vi "Generate Linear Accel Segment.vi"(0 "Speeds in":T1={"maxV (fps)"=20.0, "Accel Limit (fps^2)"=20.0, "Initial V (fps)"=0.0, "Sample Period (s)"=0.02, "Jerk Limit (fps^3)"=0.0, "Distances"=[]}, 1 "Initial Acceleration":dbl format="%#_13g", 5 "Stoopid V":dbl=20.0, 7 "Velocities":dbl[](array[numeric]), 9 "Linear Info":T2, 11 "Max Robot Speed":dbl format="%#_13g", 12 "Index":i32, 14 "Stoopid Overlap distance":dbl min=0.0) -> (3 "Final Acceleration":dbl, 4 "Speeds out":T1={"maxV (fps)"=20.0, "Accel Limit (fps^2)"=20.0, "Initial V (fps)"=0.0, "Sample Period (s)"=0.02, "Jerk Limit (fps^3)"=0.0, "Distances"=[]}, 6 "Trajectory Segment":T3, 10 "Final Position":cluster{dbl, dbl, dbl}, 15 "Valid":bool)   [LabVIEW 2025]
uses:
  Types/Speeds.ctl
panel:
  out "Waveform Graph":dbl[][](graph)
  out "XY Graph":cluster{dbl, dbl}[](graph)
  out "Segment Time (s)":dbl
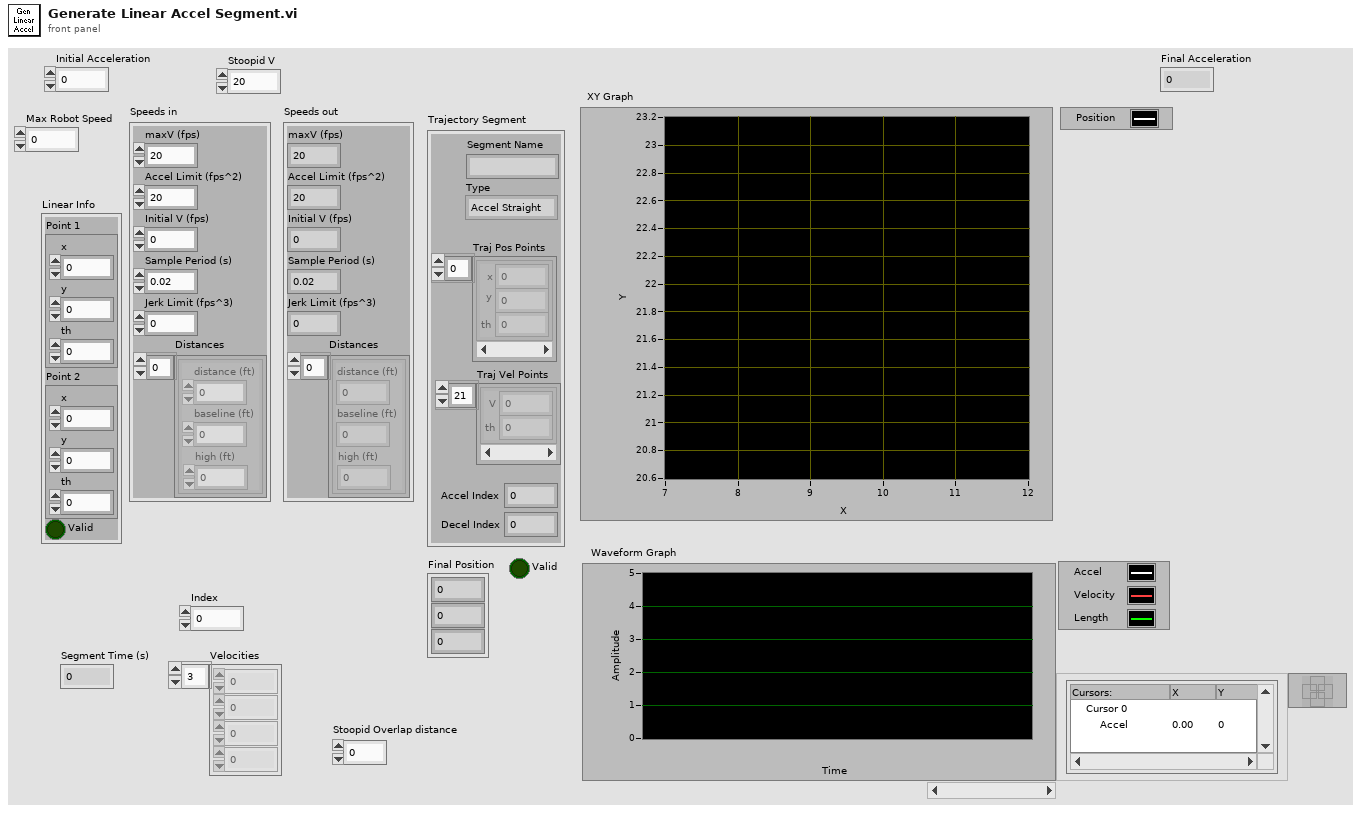
[diagram p1: front panel]
types:
  T1 = typedef "Speeds.ctl" = cluster{"maxV (fps)":dbl, "Accel Limit (fps^2)":dbl, "Initial V (fps)":dbl, "Sample Period (s)":dbl, "Jerk Limit (fps^3)":dbl, "Distances":cluster{"distance (ft)":dbl, "baseline (ft)":dbl, "high (ft)":dbl}[]}
  T2 = cluster{"Point 1":cluster{"x":dbl, "y":dbl, "th":dbl}, "Point 2":cluster{"x":dbl, "y":dbl, "th":dbl}, "Valid":bool}
  T3 = cluster{"Segment Name":string, "Type":enum16{"Accel Straight", "Const Straight", "Blend", "Circle"}, "Traj Pos Points":cluster{"x":dbl, "y":dbl, "th":dbl}[], "Traj Vel Points":cluster{"V":dbl, "th":dbl}[], "Accel Index":i32, "Decel Index":i32}
  T4 = enum16{"Accel Straight", "Const Straight", "Blend", "Circle"}
  T5 = cluster{"Accel Limit (fps^2)":dbl, "Jerk Limit (fps^3)":dbl}
  T6 = cluster{"distance (ft)":dbl, "dist baseline jerk":dbl, "dist of high Jerk":dbl}[]
  T7 = cluster{"Initial Acceleration":dbl, "Initial V (fps)":dbl}
  T8 = cluster{string, "Type":enum16{"Accel Straight", "Const Straight", "Blend", "Circle"}, cluster{dbl, dbl, dbl}[], cluster{"velocity":dbl, dbl}[], "Accel Index":i32, "Decel Index":i32}
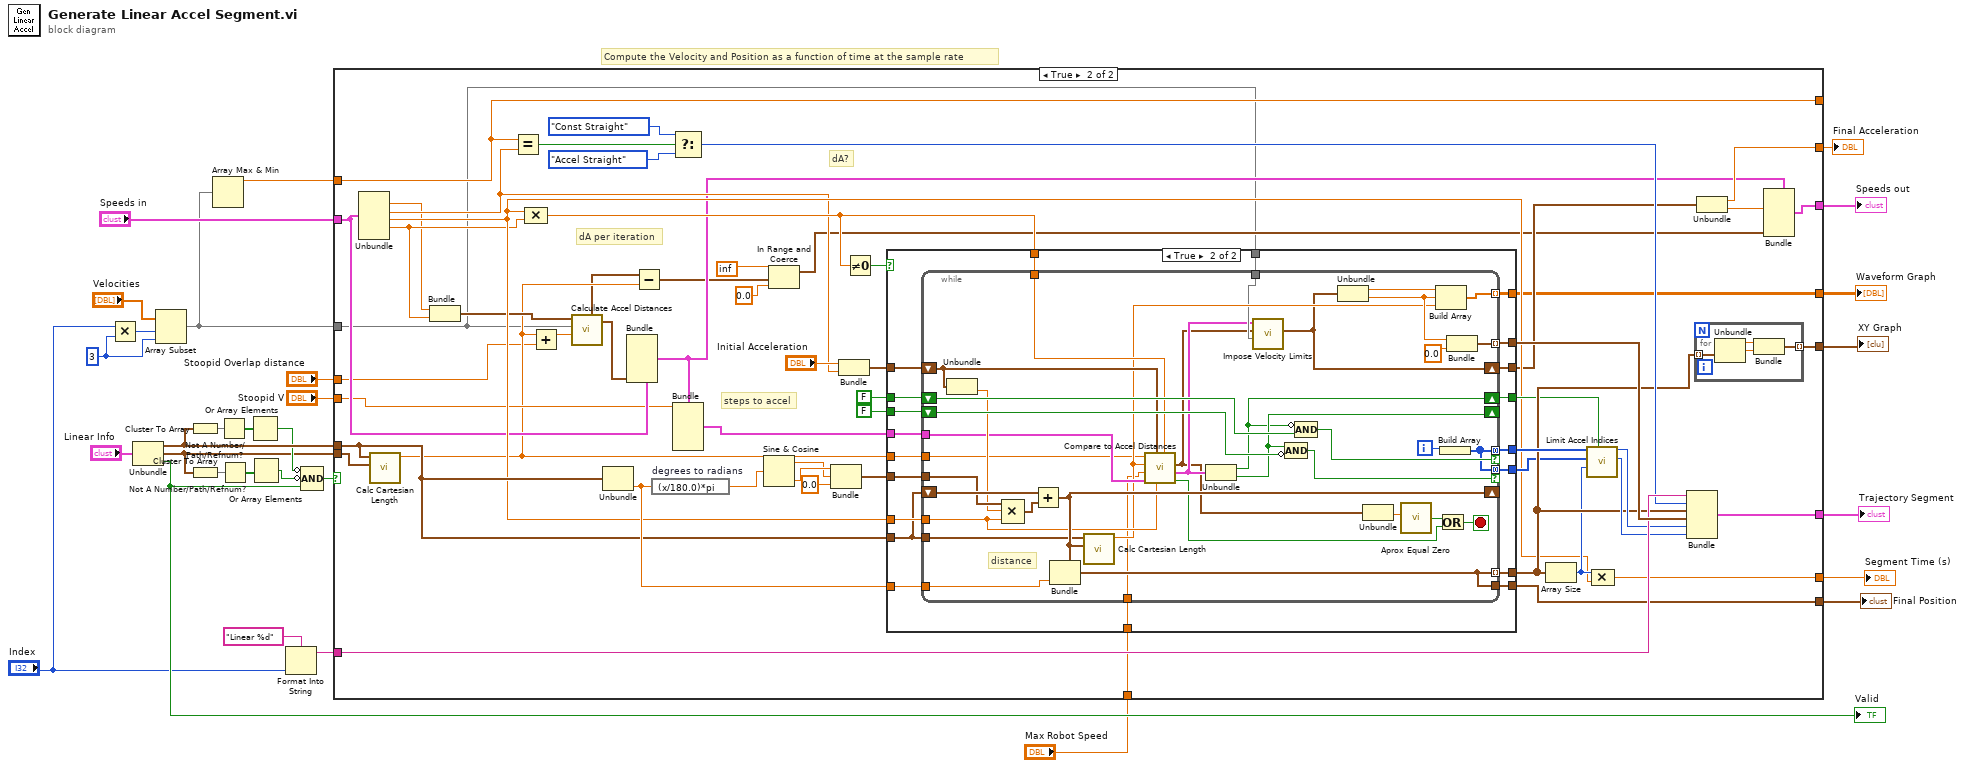
[diagram p0: block diagram]
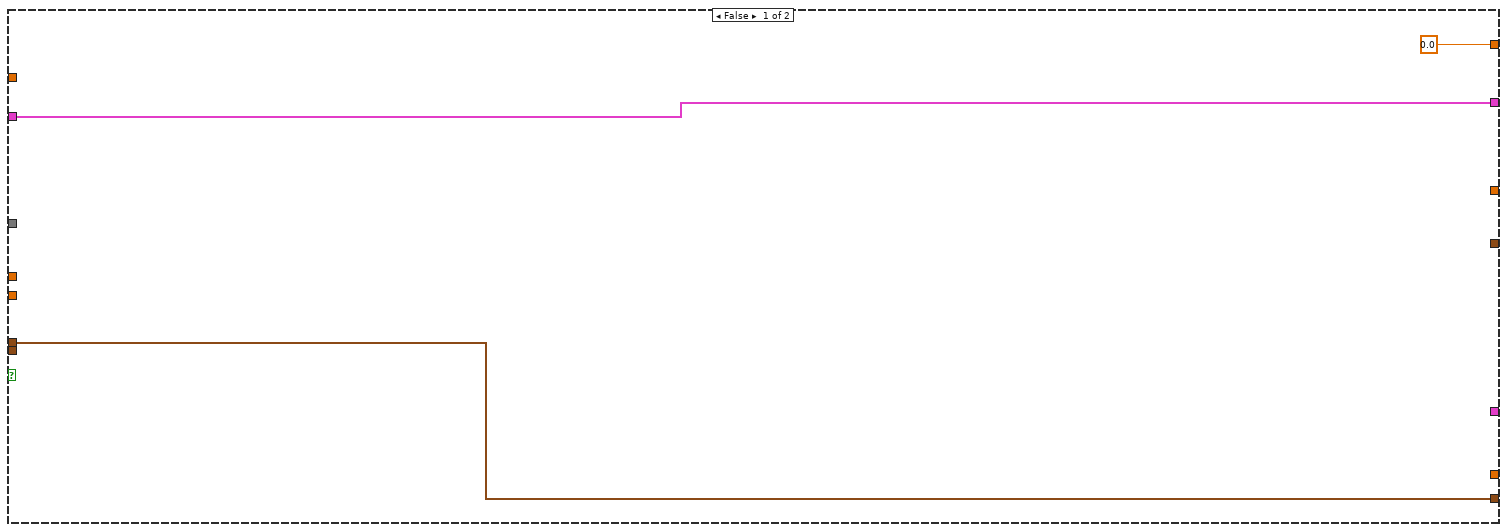
[diagram p2: hidden frame]
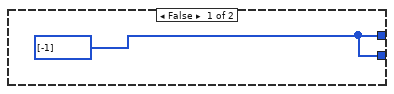
[diagram p3: hidden frame]
diagram:
  w7 = 3
  # "Compute the Velocity and Position as a function of time at the sample rate"
  n1 = Multiply(x="Index", y=w7) -> (x*y=w9:i32)
  n2 = Unbundle("Linear Info") -> ("Point 1"=w19:cluster{"x":dbl, "y":dbl, "th":dbl}, "Point 2"=w14:cluster{"x":dbl, "y":dbl, "th":dbl}, "Valid"=w20:bool)
  "Valid" <- w20
  n3 = Array Subset(array="Velocities", index=w9, length=w7) -> (w5:dbl[])
  n4 = Cluster To Array(cluster=w19) -> (array=w18:dbl[])
  n5 = Cluster To Array(cluster=w14) -> (array=w15:dbl[])
  n6 = Array Max & Min(array=w5) -> (max value=w4:dbl)  [unwired: 3 out]
  n7 = Not A Number/Path/Refnum?(number/path/refnum=w18) -> (NaN/Path/Refnum?=w17:bool[])
  n8 = Not A Number/Path/Refnum?(number/path/refnum=w15) -> (NaN/Path/Refnum?=w13:bool[])
  n9 = Or Array Elements(Boolean array=w17) -> (logical OR=w16:bool)
  n10 = Or Array Elements(Boolean array=w13) -> (logical OR=w12:bool)
  n11 = Format Into String(format string="Linear %d", "Index") -> (resulting string=w22:string)  [unwired: 2 in, 1 out]
  n12 = Compound Arithmetic op=AND(invert w16, invert w12, w20) -> (w21:bool)
  n13 = case shown="True" w21 {
    tunnel: [_ w90] -> w30
    tunnel: w22 -> [_ w84]
    tunnel: [_ w80] -> w29
    tunnel: [w32 w79] -> w28
    tunnel: [_ w76] -> w27
    tunnel: "Speeds in" -> [w33 w49]
    tunnel: [w33 w75] -> w25
    tunnel: w19 -> [w32 w70]
    tunnel: w14 -> [_ w73]
    tunnel: [_ w54] -> w11
    tunnel: [0.0 w53] -> w10
    tunnel: w5 -> [_ w35]
    tunnel: w4 -> [_ w48]
    tunnel: "Stoopid V" -> [_ w45]
    tunnel: [_ w48] -> _
    tunnel: "Stoopid Overlap distance" -> [_ w39]
    tunnel: "Max Robot Speed" -> [_ w34]
    frame False {
    }
    frame True {
      # "dA?"
      # "steps to accel"
      # "dA per iteration"
      n14 = Unbundle(w49) -> ("Accel Limit (fps^2)"=w51:dbl, "Initial V (fps)"=w58:dbl, "Sample Period (s)"=w60:dbl, "Jerk Limit (fps^3)"=w52:dbl)  [unwired: 2 out]
      n15 = call "Calc Cartesian Length.vi"("Point 2"=w73, "Point 1"=w70) -> ("Length (f)"=w44:dbl)  [unwired: 8 in, 1 out]
      n16 = Bundle("Accel Limit (fps^2)"=w51, "Jerk Limit (fps^3)"=w52) -> (w50:T5)  [unwired: 1 in]
      n17 = Equal?(x=w48, y=w58) -> (x = y?=w74:bool)
      n18 = Compound Arithmetic op=MULTIPLY(w60, w52) -> (w72:dbl)
      n19 = Add(x=w44, y=w39) -> (x+y=w38:dbl)
      n20 = call "Calculate Accel Distances.vi"("Length (f)"=w38, "Velocities"=w35, "Limits"=w50) -> ("Distances"=w37:T6, "Const V Dist"=w36:T6)  [unwired: 7 in]
      n21 = Unbundle(w70) -> ("th"=w78:dbl)  [unwired: 2 out]
      n22 = Bundle(cluster=w49, "Distances"=w37) -> (w47:T1)  [unwired: 5 in]
      n23 = Subtract(x=w36, y=w44) -> (x-y=w41:T6)
      n24 = expression code="(x/180.0)*pi" "degrees to radians"(w78) -> (w77:dbl)
      n25 = Select(t=T4."Const Straight" ("Type"), s=w74, f=T4."Accel Straight" ("Type")) -> (s? t:f=w81:T4)
      n26 = Bundle(cluster=w47, "maxV (fps)"=w45) -> (w46:T1)  [unwired: 5 in]
      n27 = Sine & Cosine(0:w77) -> (1:w85:dbl, 2:w86:dbl)
      n28 = In Range and Coerce(upper limit=inf, x=w41, lower limit=0.0) -> (coerced(x)=w40:T6)  [unwired: 1 out]
      n29 = Bundle(w86, w85, 0.0) -> (w88:cluster{dbl, dbl, dbl})  [unwired: 1 in]
      n30 = Bundle("Initial Acceleration"="Initial Acceleration", "Initial V (fps)"=w58) -> (w57:T7)  [unwired: 1 in]
      n31 = Not Equal To 0?(x=w72) -> (x != 0?=w71:bool)
      n32 = case shown="True" w71 {
        tunnel: [_ w115] -> w89
        tunnel: w88 -> [_ w114]
        tunnel: [_ w113] -> w79
        tunnel: w78 -> [_ w112]
        tunnel: [_ w111] -> w64
        tunnel: [_ w110] -> w56
        tunnel: w72 -> [_ w109]
        tunnel: w60 -> [_ w108]
        tunnel: w70 -> [_ w107]
        tunnel: FALSE -> [_ w106]
        tunnel: [w95 w105] -> w67
        tunnel: w46 -> [_ w104]
        tunnel: FALSE -> [_ w103]
        tunnel: [w95 w102] -> w63
        tunnel: [_ w101] -> w61
        tunnel: w57 -> [_ w100]
        tunnel: [_ w99] -> w54
        tunnel: w44 -> [_ w98]
        tunnel: w35 -> [_ w97]
        tunnel: w34 -> [_ w96]
        frame False {
          w95 = i32[] [-1]
        }
        frame True {
          n33 = while {
            tunnel: [w143] -> w111 mode=indexing
            tunnel: w109 -> [w130]
            shift-right: [w117] -> w110
            shift-left: w100 -> [w133]
            tunnel: [w149] -> w115 mode=indexing
            tunnel: w108 -> [w127]
            tunnel: w114 -> [w147]
            tunnel: w112 -> [w150]
            tunnel: [w143] -> w113
            shift-right: [w145] -> _
            shift-left: w107 -> [w148]
            tunnel: w107 -> [w144]
            shift-right: [w129] -> w101
            shift-left: w106 -> [w141]
            tunnel: [w138] -> w105 mode=concatenating if=w140
            tunnel: w104 -> [w126]
            shift-right: [w132] -> _
            shift-left: w103 -> [w139]
            tunnel: [w138] -> w102 mode=concatenating if=w137
            tunnel: [w128] -> w99 mode=indexing
            tunnel: w98 -> [w122]
            tunnel: w97 -> [w120]
            tunnel: w96 -> [w116]
            i -> [w142]
            stop <- w136 stop-if-true
            # "distance"
            n34 = Unbundle(w133) -> ("Initial V (fps)"=w134:dbl)  [unwired: 1 out]
            n35 = Compound Arithmetic op=MULTIPLY(w147, w134, w127) -> (w146:cluster{dbl, dbl, dbl})
            n36 = Add(x=w148, y=w146) -> (x+y=w145:cluster{dbl, dbl, dbl})
            n37 = Bundle(cluster=w145, w150) -> (w143:cluster{dbl, dbl, dbl})  [unwired: 2 in]
            n38 = call "Calc Cartesian Length.vi"("Point 2"=w145, "Point 1"=w144) -> ("Length (f)"=w123:dbl)  [unwired: 8 in, 1 out]
            n39 = call "Compare to Accel Distances.vi"("dA"=w130, "Sample Period (s)"=w127, "Values"=w133, "Speeds in"=w126, "Max Robot Speed"=w116, "Current  Length"=w123, "Total Segment Length"=w122) -> ("End Loop"=w121:bool, "Ends"=w119:cluster{"Accel End":bool, "Decel End":bool}, "Values out"=w118:cluster{"accel":dbl, "velocity":dbl})  [unwired: 1 in, 1 out]
            n40 = Unbundle(w119) -> ("Accel End"=w129:bool, "Decel End"=w132:bool)
            n41 = call "Impose Velocity Limits.vi"("Array"=w120, "Values in"=w118, "Ends"=w119) -> ("Values out"=w117:cluster{"accel":dbl, "velocity":dbl})  [unwired: 8 in]
            n42 = Compound Arithmetic op=AND(w132, invert w139) -> (w137:bool)
            n43 = Compound Arithmetic op=AND(invert w129, w141) -> (w140:bool)
            n44 = Unbundle(w117) -> ("accel"=w124:dbl, "velocity"=w125:dbl)
            n45 = Unbundle(w118) -> ("velocity"=w131:dbl)  [unwired: 1 out]
            n46 = call "Aprox Equal Zero.vi"("x"=w131) -> ("Boolean"=w135:bool)  [unwired: 10 in]
            n47 = Build Array(w124, w125, w123) -> (w128:dbl[])
            n48 = Or(x=w135, y=w121) -> (x .or. y?=w136:bool)
            n49 = Build Array(w142) -> (w138:i32[])
            n50 = Bundle("velocity"=w125, 0.0) -> (w149:cluster{"velocity":dbl, dbl})  [unwired: 1 in]
          }
        }
      }
      n51 = Array Size(array=w64) -> (size(s)=w62:i32)
      n52 = call "Limit Accel Indices.vi"("Last Accel"=w61, "Size"=w62, "Decel"=w63, "Accel"=w67) -> ("Decel Index"=w66:i32, "Accel Index"=w68:i32)  [unwired: 6 in]
      n53 = Compound Arithmetic op=MULTIPLY(w62, w60) -> (w80:dbl)
      n54 = Bundle(w84, "Type"=w81, w64, w89, "Accel Index"=w68, "Decel Index"=w66) -> (w90:T8)  [unwired: 1 in]
      n55 = for {
        tunnel: w64 -> [w94] mode=indexing
        tunnel: [w91] -> w76 mode=indexing
        n56 = Unbundle(w94) -> (w93:dbl, w92:dbl)  [unwired: 1 out]
        n57 = Bundle(w93, w92) -> (w91:cluster{dbl, dbl})  [unwired: 1 in]
      }
      n58 = Unbundle(w56) -> ("Initial Acceleration"=w53:dbl, "Initial V (fps)"=w55:dbl)
      n59 = Bundle(cluster=w47, "Initial V (fps)"=w55, "Distances"=w40) -> (w75:T1)  [unwired: 4 in]
    }
  }
  "Trajectory Segment" <- w30
  "Segment Time (s)" <- w29
  "Final Position" <- w28
  "XY Graph" <- w27
  "Speeds out" <- w25
  "Waveform Graph" <- w11
  "Final Acceleration" <- w10
